vi "Write Ready and Wait.vi"(0 "File Directory":path, 11 "error in (no error)":errorcluster) -> (4 "Stop?":bool, 6 "Exit?":bool, 15 "error out":errorcluster)   [LabVIEW 2014]
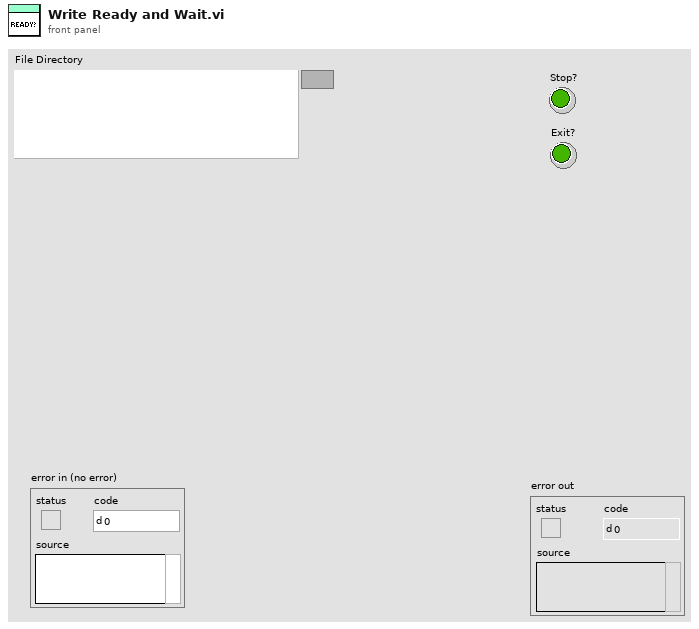
[diagram p1: front panel]
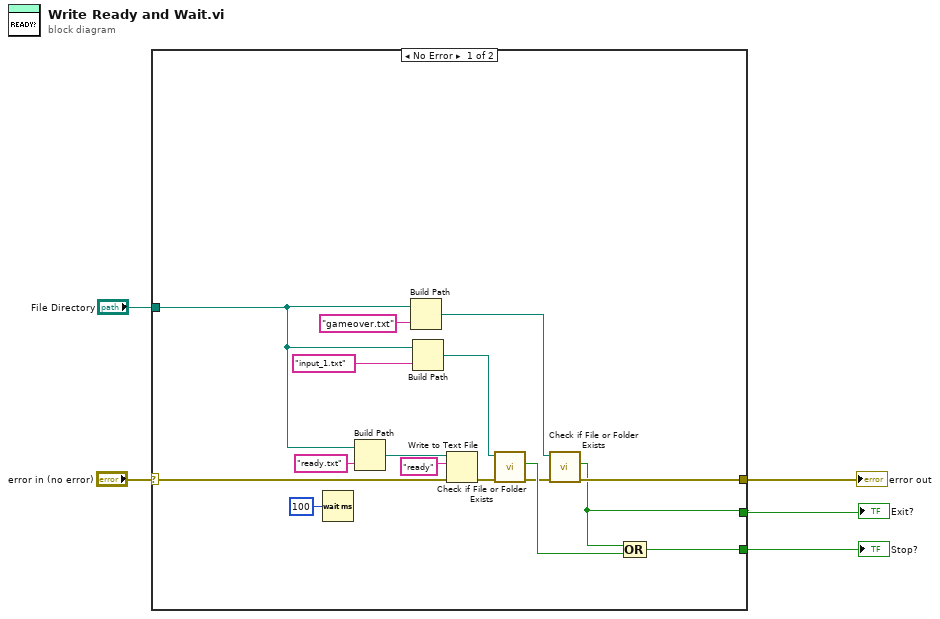
[diagram p0: block diagram]
diagram:
  n1 = case shown="No Error" "error in (no error)" {
    selector: "error in (no error)" -> [w21 w22]
    tunnel: [w20 w22] -> w4
    tunnel: "File Directory" -> [w19 _]
    tunnel: [w18 _] -> w2
    tunnel: [w6 _] -> w1
    frame No Error {
      n2 = Wait (ms)(milliseconds to wait=u32 100) -> ()  [unwired: 1 out]
      n3 = Build Path(base path=w19, name or relative path="ready.txt") -> (appended path=w11:path)
      n4 = Build Path(base path=w19, name or relative path="gameover.txt") -> (appended path=w9:path)
      n5 = Build Path(base path=w19, name or relative path="input_1.txt") -> (appended path=w15:path)
      n6 = Write to Text File(file (use dialog)=w11, text="ready", error in=w21) -> (error out=w17:errorcluster)  [unwired: 1 in, 2 out]
      n7 = call <vilib>:"Check if File or Folder Exists.vi"("error in (no error)"=w17, "path"=w15) -> ("error out"=w8:errorcluster, "file or folder exists?"=w13:bool)  [unwired: 7 in, 1 out]
      n8 = call <vilib>:"Check if File or Folder Exists.vi"("error in (no error)"=w8, "path"=w9) -> ("error out"=w20:errorcluster, "file or folder exists?"=w18:bool)  [unwired: 7 in, 1 out]
      n9 = Compound Arithmetic op=OR(w18, w13) -> (w6:bool)
    }
    frame Error {
    }
  }
  "error out" <- w4
  "Exit?" <- w2
  "Stop?" <- w1
